vi "3motorDriveTest.vi"() -> ()   [LabVIEW 2019]
uses:
  <vilib>/Platform/TimedLoop/XDataNode/timing_clust.ctl
  <vilib>/Platform/TimedLoop/XDataNode/nitl_modes.ctl
  <vilib>/Platform/TimedLoop/XDataNode/wakeup.ctl
  <vilib>/Platform/TimedLoop/XDataNode/XDataNode.xnode
  builds/KNRm_ReMi_Toolkit/KNRm/KNRm_ReMi_OS6/home/lvuser/natinst/bin/KNRm_ReMi_OS6.lvlibp
  <vilib>/Platform/TimedLoop/XDataNode/XDNodeRunTimeDep.lvlib
panel:
  in  "scale":dbl
  out "ENC (deg)":dbl[](array[numeric])
  out "2keySpeed":i8
  in  "Stop Button":bool
  out "Finished Late? [i-1]":bool
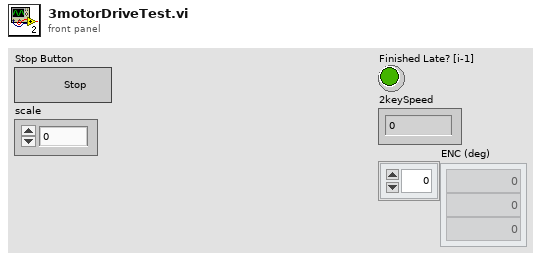
[diagram p1: front panel]
types:
  T1 = typedef "XDNodeRunTimeDep.lvlib/timing_clust.ctl" = cluster{"Expected End [f-1]":u64, "Actual End [f-1]":u64, "Finished Late? [f-1]":bool, "Expected End [i-1]":u64, "Actual End [i-1]":u64, "Finished Late? [i-1]":bool, "Expected Start [i]":u64, "Actual Start [i]":u64, "Expected Start [f]":u64, "Actual Start [f]":u64, "Source Name":string, "Structure Name":string, "Period":i64, "Deadline":i64, "Offset":i64, "Start":i64, "Priority":i32, "Timeout":i32, "Mode":T2, "Wakeup Reason":T3, "Error":errorcluster, "Source Type":string, "Secondary Source Type":string, "Global End Time":u64, "Global Start Time":u64, "Frame Duration":u64, "Iteration Duration":u64, "Assigned CPU":i32, "I/O Scan Engine Mode":u32}
  T2 = typedef "XDNodeRunTimeDep.lvlib/nitl_modes.ctl" = enum32{"No Change", "Process missed periods, maintain original phase", "Discard missed periods, maintain original phase", "Process missed periods, ignore original phase", "Discard missed periods, ignore original phase"}
  T3 = typedef "XDNodeRunTimeDep.lvlib/wakeup.ctl" = enum32{"Normal", "Aborted", "Asynchronous wakeup", "Timing source error", "Timed loop error", "Timeout"}
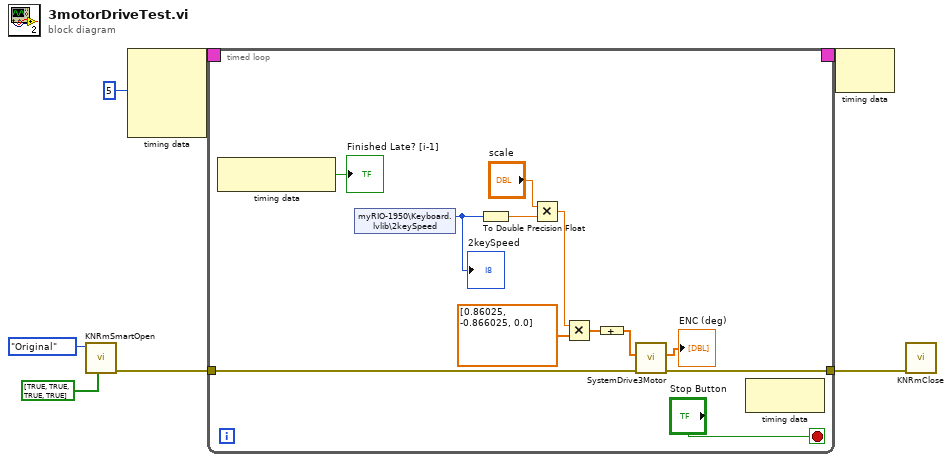
[diagram p0: block diagram]
diagram:
  n1 = call "KNRmSmartOpen.vi"("DS1-4 Mode (T: Speed/ F: PWM)"=bool[] [TRUE, TRUE, TRUE, TRUE] ("SpeedMode"), "INI FPGA MODE"=enum16{"Original", "M4EXTIOB"}."Original") -> ("error out"=w4:errorcluster)  [unwired: 6 in, 3 out]
  n2 = node-c288(i64 5 ("Period")) -> (w7:T1)  [unwired: 3 in]
  n3 = timed-loop {
    timing: w7 -> [_]
    timing-out: [_] -> w6
    tunnel: w4 -> [w17]
    tunnel: [w16] -> w2
    stop <- "Stop Button" stop-if-true
    n4 = node-c288() -> (→"Finished Late? [i-1]":bool)  [unwired: 1 in]
    n5 = shared-variable "myRIO-1950\\Keyboard.lvlib\\2keySpeed"() -> (w15:i8)  [unwired: 1 in, 1 out]
    "2keySpeed" <- w15
    n6 = To Double Precision Float(number=w15) -> (double precision float=w11:dbl)
    n7 = Multiply(x="scale", y=w11) -> (x*y=w9:dbl)
    n8 = Multiply(x=w9, y=dbl[] [0.86025, -0.866025, 0.0] ("3xMotor(deg/s)")) -> (x*y=w13:dbl[])
    n9 = Compound Arithmetic op=ADD(w13) -> (w8:dbl[])
    n10 = call "SystemDrive3Motor.vi"("error in"=w17, "3xMotor(deg/s)"=w8) -> ("error out"=w16:errorcluster, "ENC (deg)"=→"ENC (deg)":dbl[])  [unwired: 8 in]
    n11 = node-c288() -> ()  [unwired: 1 in, 1 out]
  }
  n12 = node-c288(w6) -> ()  [unwired: 1 out]
  n13 = call "KNRmClose.vi"("error in"=w2) -> ()  [unwired: 10 in, 1 out]
